vi "Run.vi"(8 "Error In":errorcluster, 11 "Lexer In":refnum<class "Lexer.lvclass">) -> (0 "Error Out":errorcluster, 2 "Tokens":refnum<class "Abstract.lvclass">[](array[class]), 3 "Lexer Out":refnum<class "Lexer.lvclass">)   [LabVIEW 2018, in "Toolkit.lvlib" / "Lexer.lvclass"]
uses:
  Lexer.lvclass
  Tokens/Abstract/Abstract.lvclass
  Lexer.lvclass/Lexer.ctl
  Support/Is Open Delimiter.vi
  Support/Pop Content.vi
  Support/Has Content.vi
  Support/Add Text Token.vi
  Support/Peek Content.vi
  Support/Is Close Delimiter.vi
  Support/Tokenize Tag.vi
  Support/Change Delimiters.vi
  Tokens/Text/Text.lvclass
  D:/Users/cfield/Code/Field R&D Services/Mustache/trunk/src/Toolkit/Low-Level/Tokens/Abstract/Abstract.lvclass
  Tokens/EscapedVariable/EscapedVariable.lvclass
  Tokens/Comment/Comment.lvclass
  Tokens/UnescapedVariable/UnescapedVariable.lvclass
  Tokens/BeginSection/BeginSection.lvclass
  Tokens/InvertedSection/InvertedSection.lvclass
  Tokens/EndSection/EndSection.lvclass
  Tokens/Partial/Partial.lvclass
  Tokens/Text/New.vi
  <vilib>/Utility/error.llb/Trim Whitespace.vi
  Tokens/EscapedVariable/New.vi
  Tokens/Comment/New.vi
  Tokens/UnescapedVariable/New.vi
  Tokens/BeginSection/New.vi
  Tokens/InvertedSection/New.vi
  Tokens/EndSection/New.vi
  Tokens/Partial/New.vi
  Readers/Abstract/Abstract.lvclass
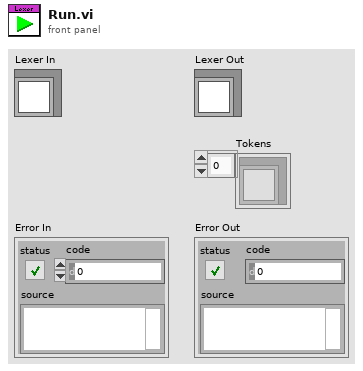
[diagram p1: front panel]
types:
  T1 = typedef "Toolkit.lvlib/Lexer.lvclass/States.ctl" = enum16{"Text", "Open Delimiter", "Tag Type", "Tag Key", "Close Delimiter"}
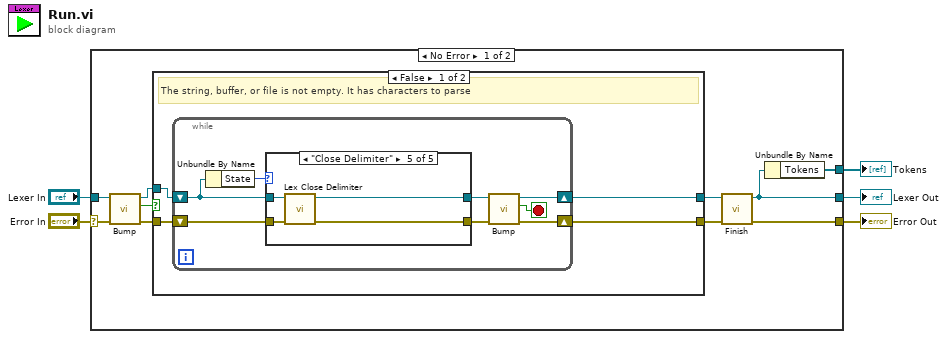
[diagram p0: block diagram]
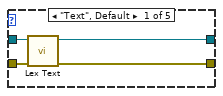
[diagram p2: hidden frame]
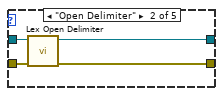
[diagram p3: hidden frame]
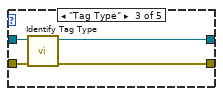
[diagram p4: hidden frame]
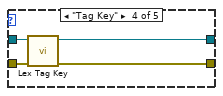
[diagram p5: hidden frame]
diagram:
  n1 = case shown="No Error" "Error In" {
    selector: "Error In" -> [w10 w50]
    tunnel: [w9 w50] -> w4
    tunnel: "Lexer In" -> [w11 _]
    tunnel: [w7 _] -> w2
    tunnel: [w6 _] -> w1
    frame No Error {
      n2 = call "Bump.vi"("Error In"=w10, "Lexer In"=w11) -> ("Error Out"=w14:errorcluster, "Done"=w13:bool, "Lexer Out"=w15:refnum<class "Lexer.lvclass">)  [unwired: 7 in]
      n3 = case shown="False" w13 {
        tunnel: [w17 w48] -> w12
        tunnel: [w16 w49] -> w8
        tunnel: w14 -> [w19 w48]
        tunnel: w15 -> [w18 w49]
        frame False {
          # "The string, buffer, or file is not empty. It has characters to parse"
          n4 = while {
            shift-right: [w21] -> w17
            shift-left: w19 -> [w25]
            shift-right: [w23] -> w16
            shift-left: w18 -> [w26]
            stop <- w22 stop-if-true
            n5 = Unbundle By Name(w26) -> ("State"=w27:T1)
            n6 = case shown="\"Close Delimiter\"" w27 {
              tunnel: w25 -> [w30 w35 w36 w40 w44]
              tunnel: w26 -> [w31 w34 w39 w43 w47]
              tunnel: [w29 w33 w38 w42 w46] -> w24
              tunnel: [w28 w32 w37 w41 w45] -> w20
              frame "Text", Default {
                n7 = call "Lex Text.vi"("Error In"=w30, "Lexer In"=w31) -> ("Error Out"=w28:errorcluster, "Lexer Out"=w29:refnum<class "Lexer.lvclass">)  [unwired: 8 in]
              }
              frame "Open Delimiter" {
                n8 = call "Lex Open Delimiter.vi"("Error In"=w35, "Lexer In"=w34) -> ("Error Out"=w32:errorcluster, "Lexer Out"=w33:refnum<class "Lexer.lvclass">)  [unwired: 8 in]
              }
              frame "Tag Type" {
                n9 = call "Identify Tag Type.vi"("Error In"=w36, "Lexer In"=w39) -> ("Error Out"=w37:errorcluster, "Lexer Out"=w38:refnum<class "Lexer.lvclass">)  [unwired: 8 in]
              }
              frame "Tag Key" {
                n10 = call "Lex Tag Key.vi"("Error In"=w40, "Lexer In"=w43) -> ("Error Out"=w41:errorcluster, "Lexer Out"=w42:refnum<class "Lexer.lvclass">)  [unwired: 8 in]
              }
              frame "Close Delimiter" {
                n11 = call "Lex Close Delimiter.vi"("Error In"=w44, "Lexer In"=w47) -> ("Error Out"=w45:errorcluster, "Lexer Out"=w46:refnum<class "Lexer.lvclass">)  [unwired: 8 in]
              }
            }
            n12 = call "Bump.vi"("Error In"=w20, "Lexer In"=w24) -> ("Error Out"=w21:errorcluster, "Done"=w22:bool, "Lexer Out"=w23:refnum<class "Lexer.lvclass">)  [unwired: 7 in]
          }
        }
        frame True {
          # "The string, buffer, file, etc. is empty. There is nothing to do."
        }
      }
      n13 = call "Finish.vi"("Error In"=w12, "Lexer In"=w8) -> ("Error Out"=w9:errorcluster, "Lexer Out"=w7:refnum<class "Lexer.lvclass">)  [unwired: 8 in]
      n14 = Unbundle By Name(w7) -> ("Tokens"=w6:refnum<class "Abstract.lvclass">[])
    }
    frame Error {
    }
  }
  "Error Out" <- w4
  "Lexer Out" <- w2
  "Tokens" <- w1
